vi "CThread Encode CThread Reference Data.vi"(4 "Clone Number":i16=-1, 5 "VI Name":string) -> (1 "CThread Reference":u32)   [LabVIEW 2012, in "CThread.lvlib"]
uses:
  CThread.lvlib
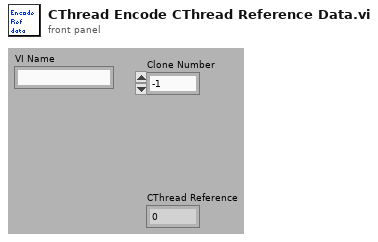
[diagram p1: front panel]
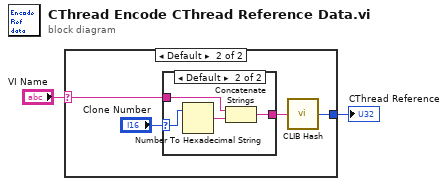
[diagram p0: block diagram]
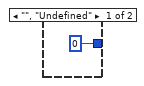
[diagram p2: hidden frame]
diagram:
  n1 = case shown="Default" "VI Name" {
    selector: "VI Name" -> [_ w6]
    tunnel: [u32 0 w7] -> w2
    frame "", "Undefined" {
    }
    frame Default {
      n2 = case shown="Default" "Clone Number" {
        selector: "Clone Number" -> [_ w10]
        tunnel: w6 -> [w8 w12]
        tunnel: [w8 w11] -> w5
        frame -1 {
        }
        frame Default {
          n3 = Number To Hexadecimal String(2:w10) -> (0:w9:string)  [unwired: 1 in]
          n4 = Concatenate Strings(w12, w9) -> (w11:string)
        }
      }
      n5 = call "CLIB Hash.vi"("Message String"=w5) -> ("32-bit Output"=w7:u32)
    }
  }
  "CThread Reference" <- w2
